vi "file_list_to_log_record.vi"(11 "cl_filename_pathout":T1(array[cluster])) -> (3 "concatenated string":string)   [LabVIEW 2026]
doc: "This subVI obtains each file name founded and generates a string"
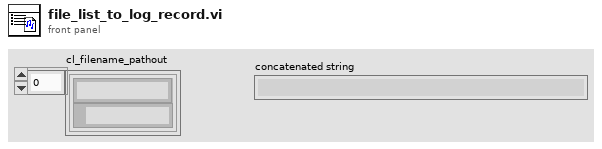
[diagram p1: front panel]
types:
  T1 = cluster{"filename":string, "arr_path out 2":path}[]
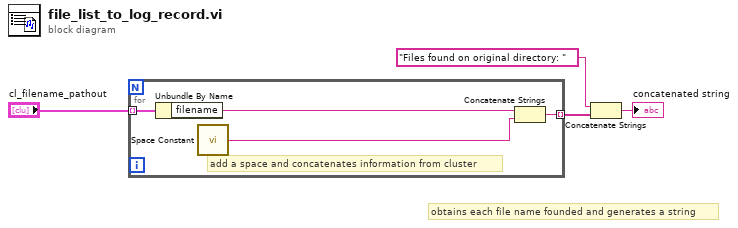
[diagram p0: block diagram]
diagram:
  # "obtains each file name founded and generates a string"
  n1 = for {
    tunnel: [w7] -> w3 mode=indexing
    tunnel: "cl_filename_pathout" -> [w6] mode=indexing
    # "add a space and concatenates information from cluster"
    n2 = Unbundle By Name(w6) -> ("filename"=w5:string)
    n3 = call <vilib>:"Space Constant.vi"() -> ("String"=w8:string)
    n4 = Concatenate Strings(w5, w8) -> (w7:string)
  }
  n5 = Concatenate Strings("Files found on original directory: ", w3) -> (→"concatenated string":string)
